vi "BRig_Host_dataRunState_typeStart_v2.vi"(5 "input_nTrial":u16, 7 "input_LorR":u16, 9 "input_idx":i32[](array[numeric]), 10 "input_dataTS":u16[][](array[numeric]), 11 "input_dataPlot":u16[][](array[numeric])) -> (1 "output_idx":i32[](array[numeric]), 2 "output_dataTS":u16[][](array[numeric]), 3 "output_dataPlot":u16[][](array[numeric]), 4 "output_updatePlot":bool)   [LabVIEW 2014]
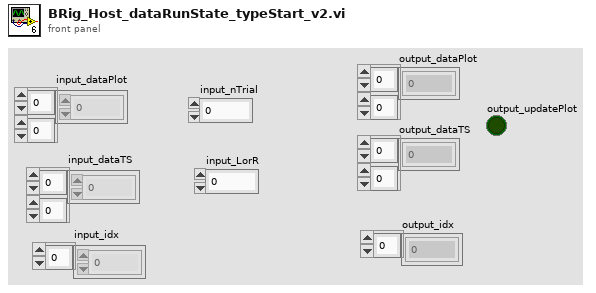
[diagram p1: front panel]
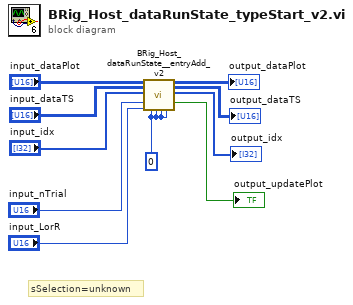
[diagram p0: block diagram]
diagram:
  w5 = u16 0 ("input_sSelection")
  # "sSelection=unknown"
  n1 = call "BRig_Host_dataRunState__entryAdd_v2.vi"("input_dataPlot"="input_dataPlot", "input_dataTS"="input_dataTS", "input_idx"="input_idx", "input_nTrial"="input_nTrial", "input_LorR"="input_LorR", "input_sSelection"=w5, "input_tSelection"=w5, "input_tSelectionPlot"=w5, "input_iSelection"=w5) -> ("output_dataPlot"=→"output_dataPlot":u16[][], "output_dataTS"=→"output_dataTS":u16[][], "output_idx"=→"output_idx":i32[], "output_updatePlot"=→"output_updatePlot":bool)  [unwired: 7 in]
